vi "Remove Subscriber.vi"(8 "error in (no error)":errorcluster, 10 "Publisher to Remove":string, 11 "CIF_CIPC_Chn in":refnum<class "CIF_CIPC_Chn.lvclass">) -> (0 "error out":errorcluster, 3 "CIF_CIPC_Chn out":refnum<class "CIF_CIPC_Chn.lvclass">)   [LabVIEW 2021, in "CIF_CIPC_Chn.lvclass"]
uses:
  CIF_CIPC_Chn.lvclass
  CIFChannels/CIFChannels.lvclass/CIFChannels.ctl
  CIF_CIPC_Chn.lvclass/CIF_CIPC_Chn.ctl
  CIFChannels/CIFChannels.lvclass
  D:/dev/Packages/CIF_Channels_Core/src/CIFChannels/CIFChannels.lvclass
  D:/dev/Packages/CIF_Channels_Core/src/CIPC_Channels/CIF_CIPC_Chan/CIF_CIPC_Chn.lvclass
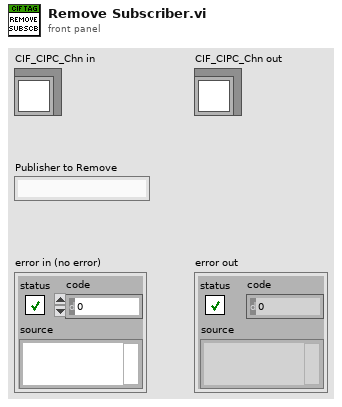
[diagram p1: front panel]
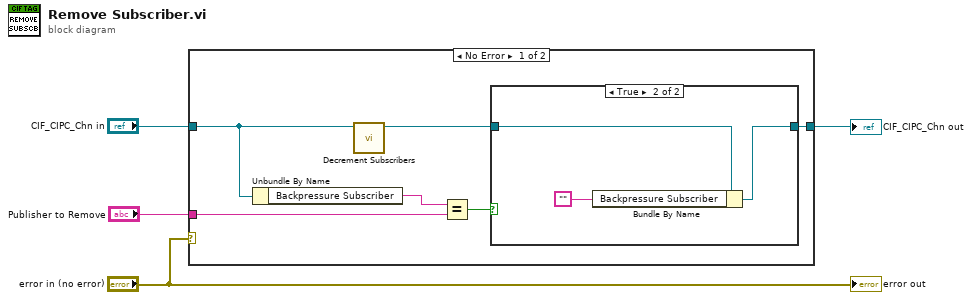
[diagram p0: block diagram]
diagram:
  n1 = case shown="No Error" "error in (no error)" {
    tunnel: "Publisher to Remove" -> [w9 _]
    tunnel: "CIF_CIPC_Chn in" -> [w6 w15]
    tunnel: [w7 w15] -> w2
    frame No Error {
      n2 = Unbundle By Name(w6) -> ("Backpressure Subscriber"=w10:string)
      n3 = call "Decrement Subscribers.vi"("CIFChannels in"=w6) -> ("CIFChannels out"=w5:refnum<class "CIF_CIPC_Chn.lvclass">)  [unwired: 9 in, 1 out]
      n4 = Equal?(x=w10, y=w9) -> (x = y?=w8:bool)
      n5 = case shown="True" w8 {
        tunnel: w5 -> [w11 w14]
        tunnel: [w11 w12] -> w7
        frame False {
        }
        frame True {
          n6 = Bundle By Name(cluster=w14, "Backpressure Subscriber"="") -> (w12:refnum<class "CIF_CIPC_Chn.lvclass">)
        }
      }
    }
    frame Error {
    }
  }
  "CIF_CIPC_Chn out" <- w2
  "error out" <- "error in (no error)"
